vi "Measure Proximity.vi"(1 "Position 1":dbl[](array[numeric]), 2 "Position 2":dbl[](array[numeric])) -> (0 "Proximity":dbl)   [LabVIEW 2017]
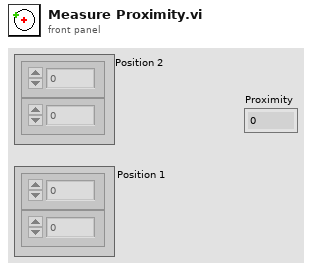
[diagram p1: front panel]
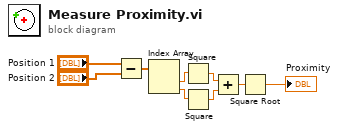
[diagram p0: block diagram]
diagram:
  n1 = Subtract(x="Position 1", y="Position 2") -> (x-y=w9:dbl[])
  n2 = Index Array(array=w9) -> (element #1=w8:dbl, element #2=w7:dbl)  [unwired: 2 in]
  n3 = Square(x=w8) -> (x^2=w5:dbl)
  n4 = Square(x=w7) -> (x^2=w6:dbl)
  n5 = Add(x=w5, y=w6) -> (x+y=w4:dbl)
  n6 = Square Root(x=w4) -> (sqrt(x)=→"Proximity":dbl)
